vi "Load ini-file.vi"(8 "error in":errorcluster, 11 "Data Cluster in":T1) -> (0 "error out":errorcluster, 3 "Data Cluster out":T1)   [LabVIEW 2022 SP3, in "hse-db.lvlib" / "DB_CONNECTOR.lvlib"]
doc: "Load the specific configuration from the ini-file.\n\n____\nHAMPEL SOFTWARE ENGINEERING v1.4.0 (2023-12-19 09:52)"
uses:
  DB_CONNECTOR.lvlib
  Module Data--cluster.ctl
  DB-Interface/DB-Interface.lvclass
  hse-libraries/Source/hse-configuration/config-base/config-base.lvclass
  hse-libraries/Source/hse-configuration/config-ini/config-ini.lvclass
  C:/Projects/579-Intelligent-Systems-Term-Project/06_Source/UI/FReVSys_Source/Libraries/hse-libraries/Source/hse-configuration/config-base/config-base.lvclass
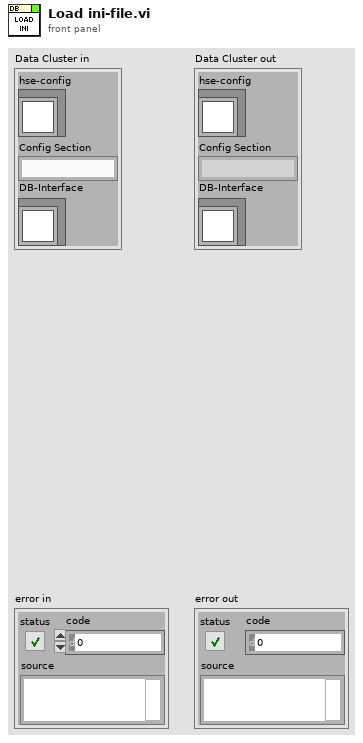
[diagram p1: front panel]
types:
  T1 = typedef "hse-db.lvlib/DB_CONNECTOR.lvlib/Module Data--cluster.ctl" = cluster{"hse-config":refnum<class "config-base.lvclass">, "Config Section":string, "DB-Interface":refnum<class "DB-Interface.lvclass">}
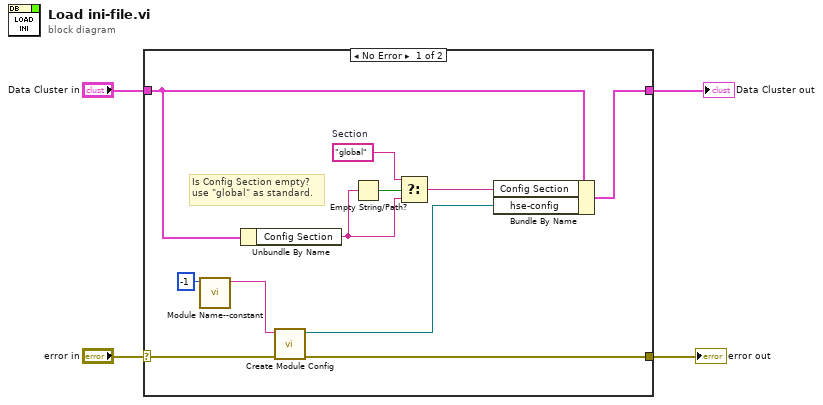
[diagram p0: block diagram]
diagram:
  n1 = case shown="No Error" "error in" {
    selector: "error in" -> [w6 w17]
    tunnel: [w5 w17] -> w4
    tunnel: [w14 w16] -> w3
    tunnel: "Data Cluster in" -> [w13 w16]
    frame No Error {
      w11 = "global"  # Section
      # "Is Config Section empty?\nuse \"global\" as standard."
      n2 = call "Module Name--constant.vi"("Module ID"=-1) -> ("Module Name"=w7:string)  [unwired: 10 in]
      n3 = Unbundle By Name(w13) -> ("Config Section"=w10:string)
      n4 = call "Create Module Config.vi"("error in"=w6, "DQMH Module Name"=w7) -> ("error out"=w5:errorcluster, "config-ini out"=w8:refnum<class "config-ini.lvclass">)  [unwired: 8 in]
      n5 = Empty String/Path?(string/path=w10) -> (empty?=w12:bool)
      n6 = Select(t=w11, s=w12, f=w10) -> (s? t:f=w9:string)
      n7 = Bundle By Name(cluster=w13, "Config Section"=w9, "hse-config"=w8) -> (w14:T1)
    }
    frame Error {
    }
  }
  "error out" <- w4
  "Data Cluster out" <- w3
